vi "DiffDriveOdom_Trajectory_Globals.vi"() -> ()   [LabVIEW 2019]
panel:
  out "Traj_RamseteEnabled":bool=TRUE
  out "Traj Samp Pose Y":dbl format="%17.2f"
  out "Traj Samp Pose X":dbl format="%17.2f"
  out "Traj Samp Curvature":dbl format="%17.2f"
  out "Traj Samp Velocity":dbl format="%17.2f"
  out "Traj Samp Accel":dbl format="%17.2f"
  out "Traj Samp Time":dbl format="%17.2f"
  out "Traj_IsGood":bool
  out "Traj_Total_Time":dbl format="%17.2f"
  out "Traj_Total_States":dbl format="%17.2f"
  out "Traj Heading Err":dbl format="%17.2f"
  out "Traj Y Err":dbl format="%17.2f"
  out "Traj X Err":dbl format="%17.2f"
  out "Traj_OnTarget":bool
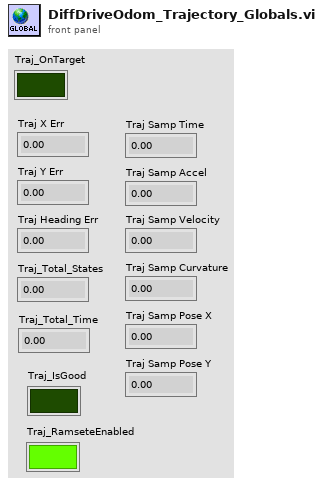
[diagram p1: front panel]
diagram:
